vi "Convert to Controller Interface State.vi"(8 "error in (no error)":errorcluster, 11 "Instrument State":T2={"Data Directory"=path "", "Last Report Number"=0, "Yield"=0.0, "Max Concentration (mM)"=1.0, "Report File Pattern"="", "Current Data File"=path "", "Peak Data Array"=[], "Average Peak Data"={"Time Stamp"=timestamp(0 s since 1904-01-01), "Peaks"=[]}, "Points to Average"=3}) -> (0 "error out":errorcluster, 3 "Analyzer State out":variant)   [LabVIEW 2020, in "Waters Patrol UPLC Report Parser.lvlib" / "Remote Connection Manager.lvlib"]
doc: "Converts the internal instrument state to the instrument state data required by the remote system."
uses:
  Remote Connection Manager.lvlib
  Instrument Manager/Instrument State.ctl
  Typedefs/Remote LC State.ctl
  Waters Patrol UPLC Report Parser.lvlib
  Instrument Manager/Instrument Manager.lvlib
panel:
  out "LC Parser State":T1
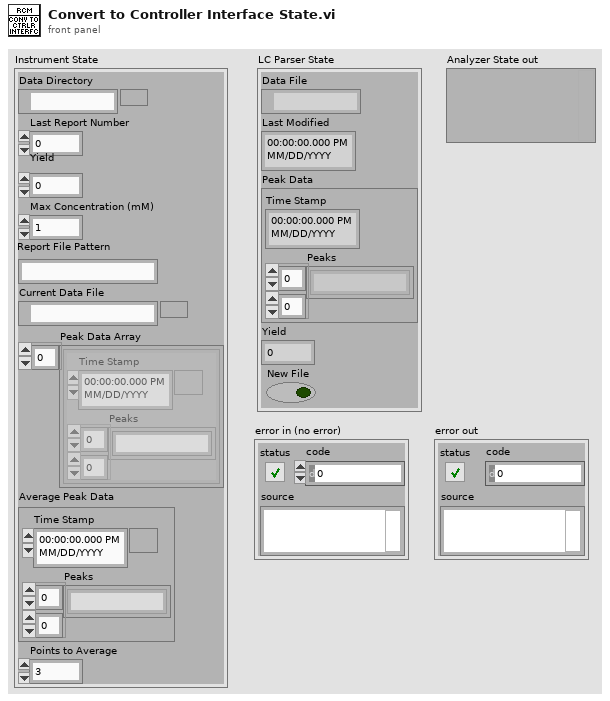
[diagram p1: front panel]
types:
  T1 = typedef "Waters Patrol UPLC Report Parser.lvlib/Remote LC State.ctl" = cluster{"Data File":path, "Last Modified":timestamp, "Peak Data":cluster{"Time Stamp":timestamp, "Peaks":string[][]}, "Yield":dbl, "New File":bool}
  T2 = typedef "Waters Patrol UPLC Report Parser.lvlib/Instrument Manager.lvlib/Instrument State.ctl" = cluster{"Data Directory":path, "Last Report Number":i32, "Yield":dbl, "Max Concentration (mM)":dbl, "Report File Pattern":string, "Current Data File":path, "Peak Data Array":cluster{"Time Stamp":timestamp, "Peaks":string[][]}[], "Average Peak Data":cluster{"Time Stamp":timestamp, "Peaks":string[][]}, "Points to Average":i32}
  T3 = cluster{"Time Stamp":timestamp, "Peaks":string[][]}[]
  T4 = cluster{"Time Stamp":timestamp, "Peaks":string[][]}
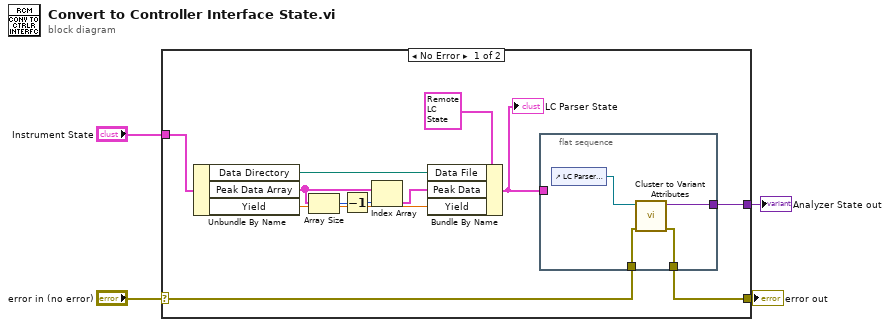
[diagram p0: block diagram]
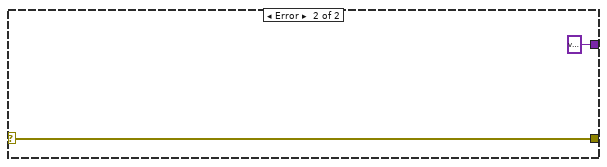
[diagram p2: hidden frame]
diagram:
  n1 = case shown="No Error" "error in (no error)" {
    selector: "error in (no error)" -> [w8 w22]
    tunnel: "Instrument State" -> [w16 _]
    tunnel: [w7 w22] -> w3
    tunnel: [w6 variant ("Variant out")] -> w1
    frame No Error {
      n2 = Unbundle By Name(w16) -> ("Data Directory"=w15:path, "Peak Data Array"=w11:T3, "Yield"=w13:dbl)
      n3 = Array Size(array=w11) -> (size(s)=w10:i32)
      n4 = Decrement(x=w10) -> (x-1=w9:i32)
      n5 = Index Array(array=w11, index=w9) -> (element=w12:T4)
      n6 = Bundle By Name(cluster=T1 {"Data File"=path "", "Last Modified"=timestamp(0 s since 1904-01-01), "Peak Data"={"Time Stamp"=timestamp(0 s since 1904-01-01), "Peaks"=[]}, "Yield"=0.0, "New File"=FALSE} ("LC Parser State"), "Data File"=w15, "Peak Data"=w12, "Yield"=w13) -> (w5:T1)
      "LC Parser State" <- w5
      n7 = flat-sequence {
        tunnel: w8 -> [w20]
        tunnel: [w19] -> w7
        tunnel: [w18] -> w6
        tunnel: w5 -> [_]
        frame #0 {
          n8 = control-ref of="LC Parser State"() -> (w17:refnum<vi>)
          n9 = call "Cluster to Variant Attributes.vi"("error in (no error)"=w20, "Cluster in"=w17) -> ("error out"=w19:errorcluster, "Variant out"=w18:variant)  [unwired: 8 in]
        }
      }
    }
    frame Error {
    }
  }
  "error out" <- w3
  "Analyzer State out" <- w1
